vi "CAN_Open.vi"(8 "error in (no error)":errorcluster caption="错误输入（无错误）", 11 "General_Input":T2) -> (0 "error out":errorcluster caption="错误输出", 2 "DeviceOpen":bool, 3 "General_Output":T1)   [LabVIEW 2012]
panel:
  in  "Reserved":u32
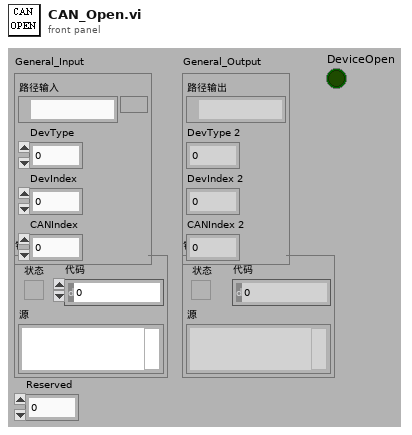
[diagram p1: front panel]
types:
  T1 = cluster{"路径输出":path, "DevType 2":u32, "DevIndex 2":u32, "CANIndex 2":u32}
  T2 = cluster{"路径输入":path, "DevType":u32, "DevIndex":u32, "CANIndex":u32}
  T3 = cluster{"path out":path, "DevType":u32, "DevIndex":u32, "CANIndex":u32}
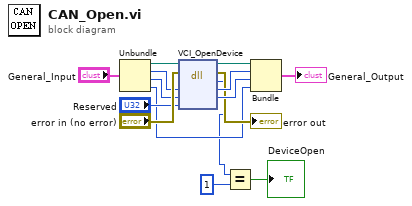
[diagram p0: block diagram]
diagram:
  n1 = Unbundle("General_Input") -> ("路径输入"=w13:path, "DevType"=w12:u32, "DevIndex"=w11:u32, "CANIndex"=w4:u32)
  n2 = dll-call lib="?" fn="VCI_OpenDevice"(path in=w13, error in="error in (no error)", "DevType"=w12, "DevIndex"=w11, "Reserved"="Reserved") -> (path out=w9:path, error out=→"error out":errorcluster, "OpenOrNot"=w3:u32, "DevType"=w8:u32, "DevIndex"=w7:u32)  [unwired: 2 in]
  n3 = Equal?(x=w3, y=u32 1) -> (x = y?=→"DeviceOpen":bool)
  n4 = Bundle("path out"=w9, "DevType"=w8, "DevIndex"=w7, "CANIndex"=w4) -> (→"General_Output":T3)  [unwired: 1 in]
